vi "WPI_DashboardAccum TCP String Buffer.vi"(10 "data in":string, 11 "string in":string) -> (2 "Array":cluster{u16, u8, "unsigned byte array":u8[]}[](array[cluster]), 3 "string out":string)   [LabVIEW 2017]
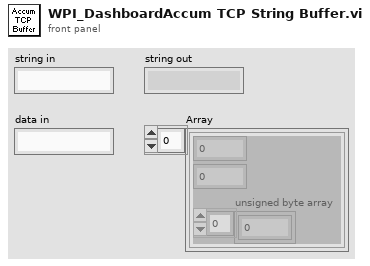
[diagram p1: front panel]
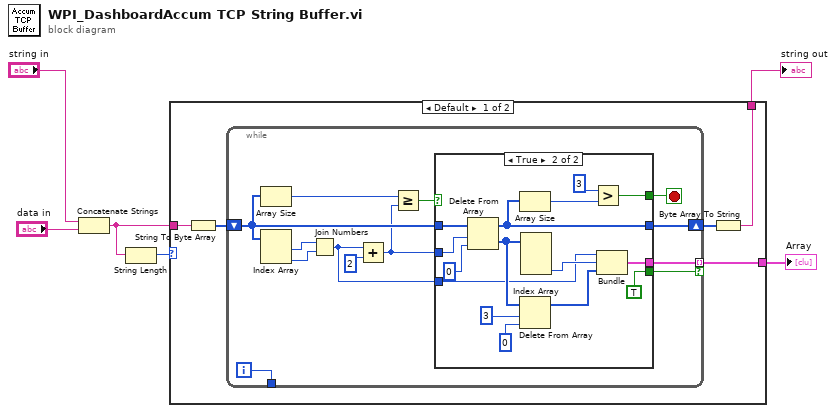
[diagram p0: block diagram]
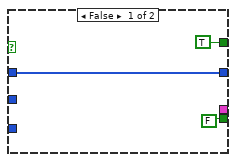
[diagram p2: hidden frame]
diagram:
  n1 = Concatenate Strings("string in", "data in") -> (w4:string)
  n2 = String Length(string=w4) -> (length=w2:i32)
  n3 = case shown="Default" w2 {
    tunnel: w4 -> [w11 w43]
    tunnel: [w9 _] -> w1
    tunnel: [w7 w43] -> w3
    frame Default {
      n4 = String To Byte Array(string=w11) -> (unsigned byte array=w10:u8[])
      n5 = while {
        shift-right: [w23] -> w8
        shift-left: w10 -> [w21]
        tunnel: [w22] -> w9 mode=indexing if=w12
        tunnel: [w17] -> _
        i -> [w17]
        stop <- w24 stop-if-true
        n6 = Array Size(array=w21) -> (size(s)=w20:i32)
        n7 = Index Array(array=w21) -> (element #1=w14:u8, element #2=w13:u8)  [unwired: 2 in]
        n8 = Join Numbers(hi=w14, lo=w13) -> ((hi.lo)=w16:u16)
        n9 = Add(x=w16, y=2) -> (x+y=w19:i32)
        n10 = Greater Or Equal?(x=w20, y=w19) -> (x >= y?=w18:bool)
        n11 = case shown="True" w18 {
          tunnel: [TRUE w37] -> w24
          tunnel: [w27 w35] -> w23
          tunnel: [_ w34] -> w22
          tunnel: w16 -> [_ w32]
          tunnel: w21 -> [w27 w30]
          tunnel: w19 -> [_ w29]
          tunnel: [FALSE TRUE] -> w12
          frame False {
          }
          frame True {
            n12 = Delete From Array(array=w30, length=w29, index=0) -> (deleted portion=w42:u8[], array with subset deleted=w35:u8[])
            n13 = Array Size(array=w35) -> (size(s)=w36:i32)
            n14 = Delete From Array(array=w42, length=3, index=0) -> (array with subset deleted=w38:u8[])  [unwired: 1 out]
            n15 = Index Array(array=w42) -> (element #3=w33:u8)  [unwired: 3 in, 2 out]
            n16 = Greater?(x=3, y=w36) -> (0:w37:bool)
            n17 = Bundle(w32, w33, "unsigned byte array"=w38) -> (w34:cluster{u16, u8, "unsigned byte array":u8[]})  [unwired: 1 in]
          }
        }
      }
      n18 = Byte Array To String(unsigned byte array=w8) -> (string=w7:string)
    }
    frame 0..2 {
    }
  }
  "string out" <- w3
  "Array" <- w1
